vi "Main.vi"() -> ()   [LabVIEW 2016]
uses:
  Type Defs/Target.ctl
  Type Defs/Current Coords.ctl
  Type Defs/Host Data.ctl
panel:
  in  "kp":dbl=0.02
  in  "kd":dbl=0.001
  in  "ki":dbl=0.002
  in  "Disturbance":bool
  out "state":string
  out "Current Position":T1
  in  "Target":T2
  in  "stop":bool
  in  "Start":bool
  in  "Tab Control":enum32{"Arm Location", "Arm Coords"}(tab)
  out "Link Picture":picture
  out "Current arm location":cluster{"X":dbl, "Y":dbl}[](graph)=[{"X"=0.0, "Y"=0.0}, {"X"=4.2862637970157365e-15, "Y"=70.0}, {"X"=70.0, "Y"=70.0}]
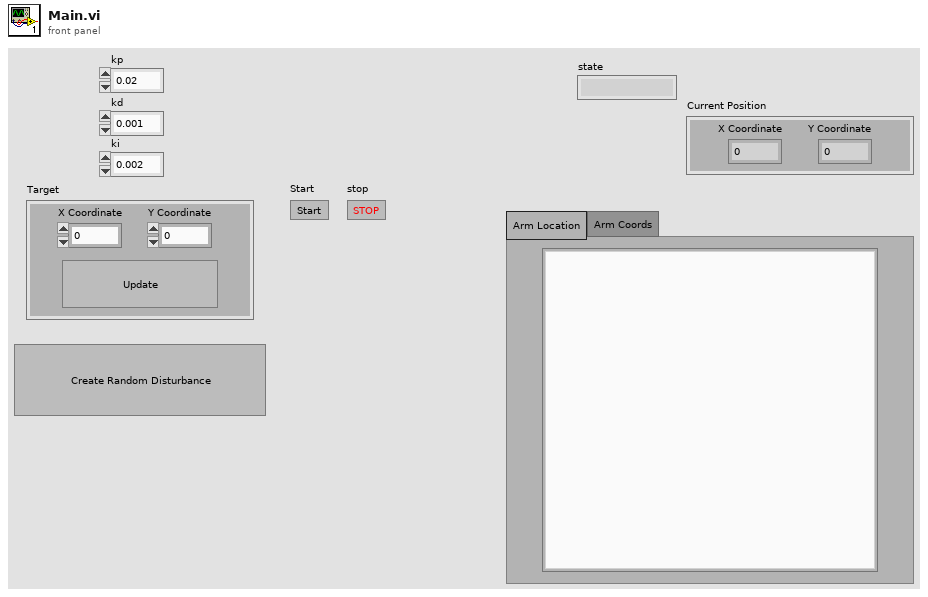
[diagram p1: front panel]
types:
  T1 = typedef "Current Coords.ctl" = cluster{"X Coordinate":dbl, "Y Coordinate":dbl}
  T2 = typedef "Target.ctl" = cluster{"X Coordinate":dbl, "Y Coordinate":dbl, "Update":bool}
  T3 = typedef "Host Data.ctl" = cluster{"link 1 angle":dbl, "link 2 angle":dbl, "link 1 length":dbl, "link 2 length":dbl, "Current arm location":cluster{"X":dbl, "Y":dbl}[], "Link Picture":picture, "Desired Location":cluster{"Desired X":dbl, "Desired Y":dbl}, "Next Location":cluster{"Next X":dbl, "Next Y":dbl}, "Error":cluster{"Joint1 error":dbl, "Joint2 error":dbl}, "tdms data":refnum<k34>, "de/dt":cluster{"joint1 de/dt":dbl, "joint2 de/dt":dbl}, "Voltages":cluster{"Joint1 voltage":dbl, "Joint2 voltage":dbl}, "Time":dbl, "dt":dbl, "counts/rev":dbl, "kp":dbl, "kd":dbl, "ki":dbl, "Int(error)":cluster{"joint1 int(e)":dbl, "joint2 int(e)":dbl}, "Desired angles":cluster{"theta 1":dbl, "theta 2":dbl}, "Current counts":cluster{"theta 1":dbl, "theta 2":dbl}, "Desired Counts":cluster{"theta 1":dbl, "theta 2":dbl}, "Preivous Error":cluster{"Joint1 Previous error":dbl, "Joint2 Previous error":dbl}, "Counts/s":dbl, "Correct counter":i32}
  T4 = enum8{"Enabled", "Disabled", "Disabled and Grayed Out"}
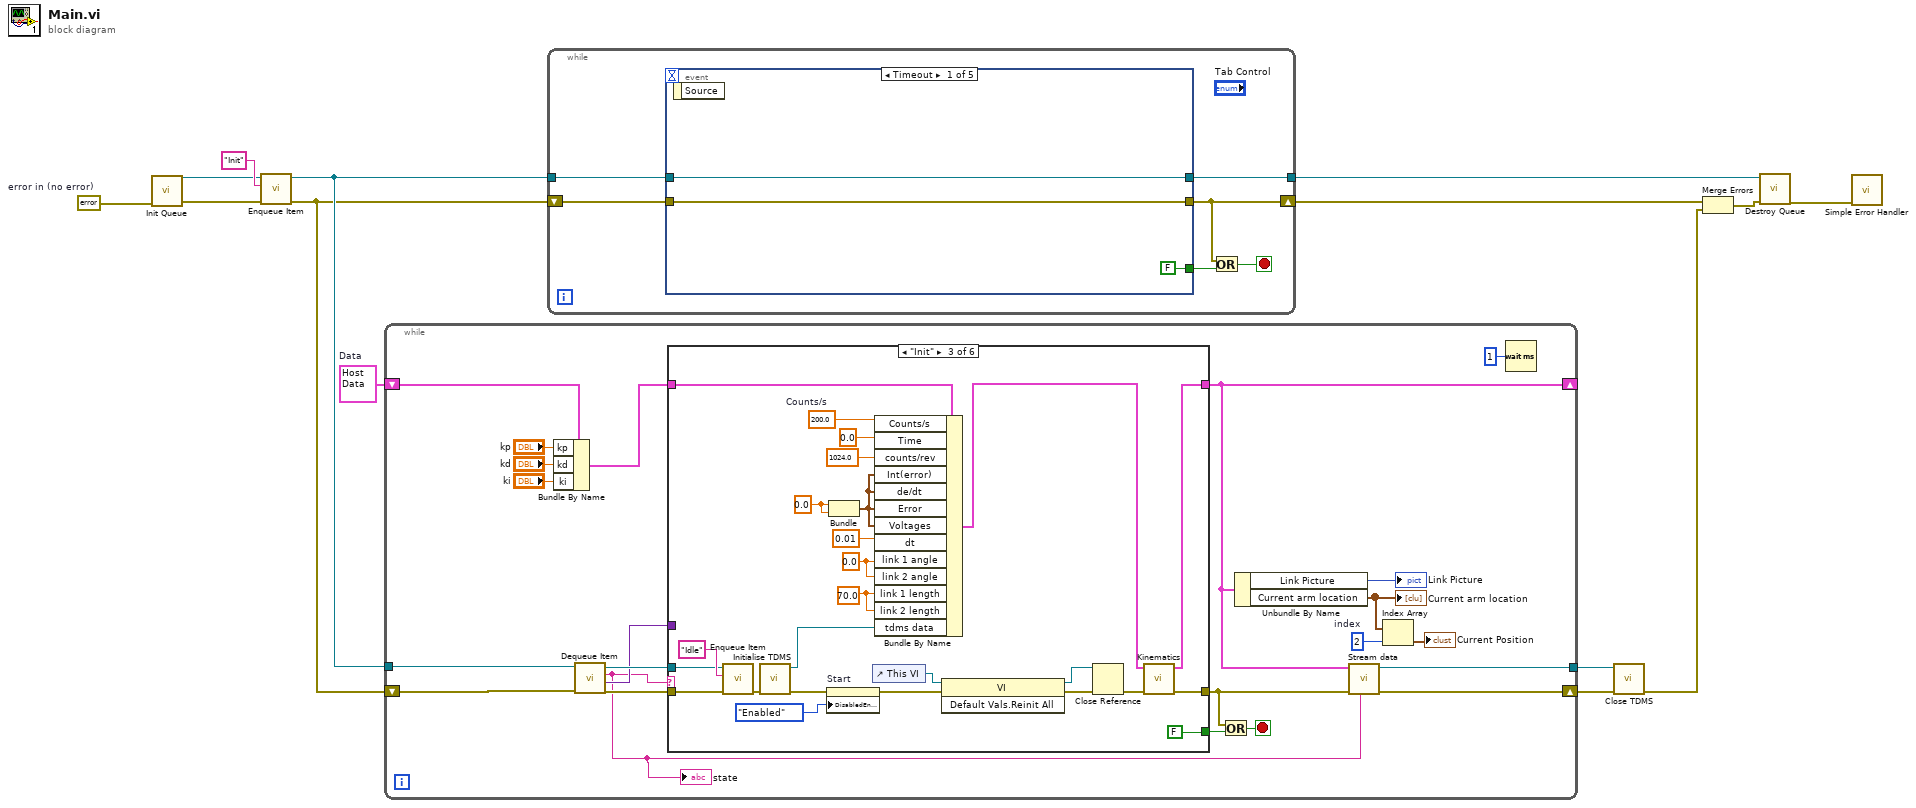
[diagram p0: block diagram]
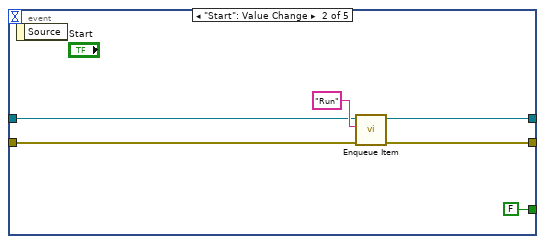
[diagram p2: hidden frame]
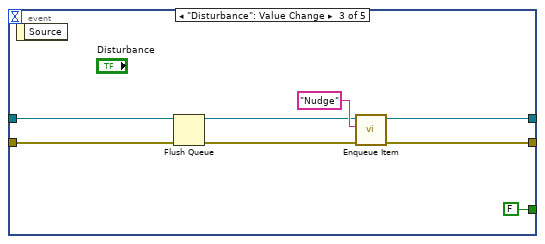
[diagram p3: hidden frame]
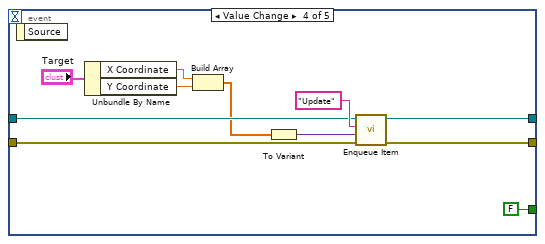
[diagram p4: hidden frame]
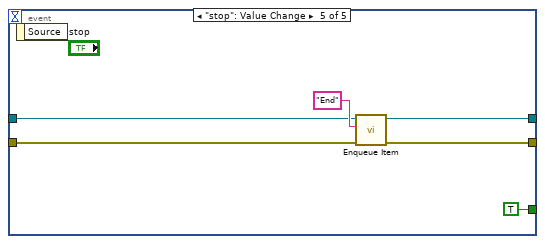
[diagram p5: hidden frame]
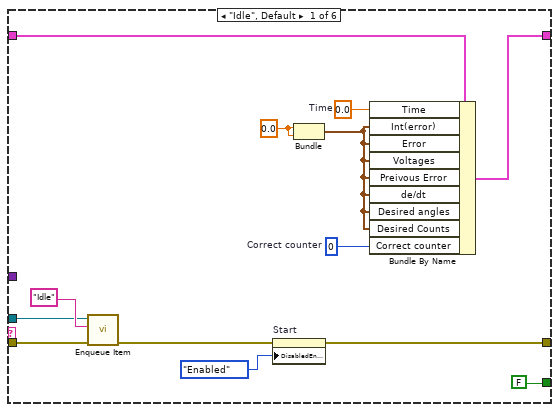
[diagram p6: hidden frame]
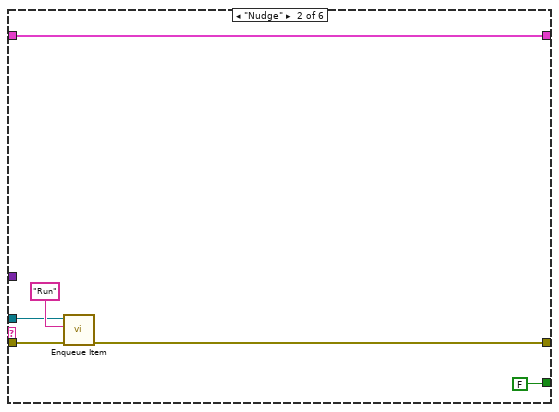
[diagram p7: hidden frame]
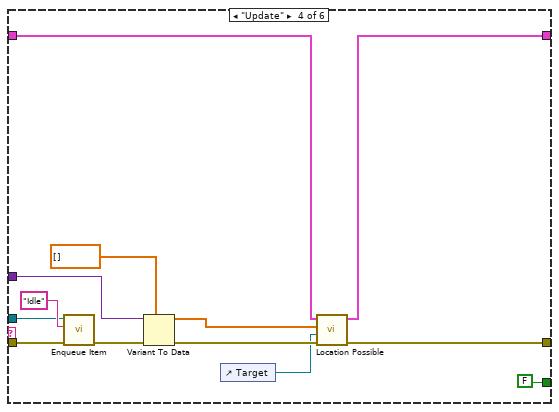
[diagram p8: hidden frame]
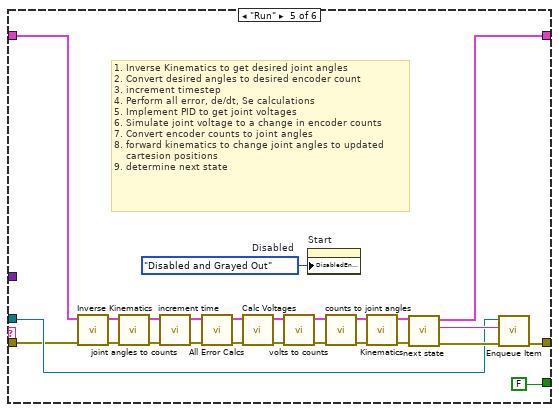
[diagram p9: hidden frame]
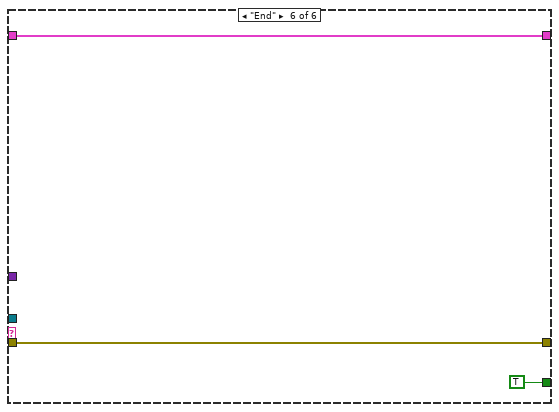
[diagram p10: hidden frame]
diagram:
  w10 = errorcluster {"status"=FALSE, "code"=0, "source"=""}  # error in (no error)
  w9 = T3 {"link 1 angle"=0.0, "link 2 angle"=0.0, "link 1 length"=0.0, "link 2 length"=0.0, "Current arm location"=[{"X"=0.0, "Y"=0.0}, {"X"=-37.249783598972314, "Y"=33.353464914904016}, {"X"=-74.49956719794463, "Y"=66.70692982980803}], "Link Picture"=bytes[1162], "Desired Location"={"Desired X"=0.0, "Desired Y"=0.0}, "Next Location"={"Next X"=0.0, "Next Y"=0.0}, "Error"={"Joint1 error"=0.0, "Joint2 error"=0.0}, "tdms data"=refnum, "de/dt"={"joint1 de/dt"=0.0, "joint2 de/dt"=0.0}, "Voltages"={"Joint1 voltage"=0.0, "Joint2 voltage"=0.0}, "Time"=0.0, "dt"=0.0, "counts/rev"=0.0, "kp"=0.0, "kd"=0.0, "ki"=0.0, "Int(error)"={"joint1 int(e)"=0.0, "joint2 int(e)"=0.0}, "Desired angles"={"theta 1"=0.0, "theta 2"=0.0}, "Current counts"={"theta 1"=0.0, "theta 2"=0.0}, "Desired Counts"={"theta 1"=0.0, "theta 2"=0.0}, "Preivous Error"={"Joint1 Previous error"=0.0, "Joint2 Previous error"=0.0}, "Counts/s"=0.0, "Correct counter"=0}  # Data
  n1 = call "Init Queue.vi"("error in (no error)"=w10) -> ("error out"=w11:errorcluster, "Queue out"=w12:refnum<queue>)  [unwired: 9 in]
  n2 = call "Enqueue Item.vi"("error in (no error)"=w11, "State"="Init", "Queue in"=w12) -> ("error out"=w4:errorcluster, "Queue out"=w13:refnum<queue>)  [unwired: 7 in]
  n3 = while {
    tunnel: w13 -> [w36]
    shift-right: [w23] -> w3
    shift-left: w4 -> [w35]
    shift-right: [w22] -> _
    shift-left: w9 -> [w19]
    tunnel: [w20] -> w1
    stop <- w31 stop-if-true
    w26 = 2  # index
    n4 = Bundle By Name(cluster=w19, "kp"="kp", "kd"="kd", "ki"="ki") -> (w18:T3)
    n5 = call "Dequeue Item.vi"("error in (no error)"=w35, "Queue in"=w36) -> ("error out"=w34:errorcluster, "Variant"=w32:variant, "String"=w21:string, "Queue out"=w33:refnum<queue>)  [unwired: 6 in]
    "state" <- w21
    n6 = case shown="\"Init\"" w21 {
      tunnel: w34 -> [w47 w53 w78 w88 w111 w121]
      tunnel: w33 -> [w46 w52 w77 w89 w113 _]
      tunnel: w32 -> [_ _ _ w93 _ _]
      tunnel: [w37 w50 w71 w81 w115 w121] -> w24
      tunnel: [FALSE FALSE FALSE FALSE FALSE TRUE] -> w30
      tunnel: w18 -> [w45 w51 w76 w85 w112 w119]
      tunnel: [w44 w51 w72 w82 w117 w119] -> w22
      frame "Idle", Default {
        w41 = 0.0 ("Time")
        w42 = 0  # Correct counter
        w43 = 0.0  # Time
        n7 = call "Enqueue Item.vi"("error in (no error)"=w47, "State"="Idle", "Queue in"=w46) -> ("error out"=w38:errorcluster)  [unwired: 7 in, 1 out]
        n8 = property on="Start" class="Bool"(error in=w38, "DisabledEnum"=T4."Enabled" ("Disabled")) -> (error out=w37:errorcluster)  [unwired: 1 in, 1 out]
        n9 = Bundle("Time"=w41, "Time"=w41) -> (w40:cluster{"Time":dbl, "Time":dbl})  [unwired: 1 in]
        n10 = Bundle By Name(cluster=w45, "Time"=w43, "Int(error)"=w40, "Error"=w40, "Voltages"=w40, "Preivous Error"=w40, "de/dt"=w40, "Desired angles"=w40, "Desired Counts"=w40, "Correct counter"=w42) -> (w44:T3)
      }
      frame "Nudge" {
        n11 = call "Enqueue Item.vi"("error in (no error)"=w53, "State"="Run", "Queue in"=w52) -> ("error out"=w50:errorcluster)  [unwired: 7 in, 1 out]
      }
      frame "Init" {
        w59 = 200.0  # Counts/s
        w64 = 0.0
        w74 = 70.0
        w75 = 0.0
        n12 = call "Enqueue Item.vi"("error in (no error)"=w78, "State"="Idle", "Queue in"=w77) -> ("error out"=w66:errorcluster)  [unwired: 7 in, 1 out]
        n13 = call "Initialise TDMS.vi"("error in (no error)"=w66) -> ("error out"=w57:errorcluster, "tdms file out"=w65:refnum<k34>)  [unwired: 9 in]
        n14 = property on="Start" class="Bool"(error in=w57, "DisabledEnum"=T4."Enabled" ("Disabled")) -> (error out=w56:errorcluster)  [unwired: 1 in, 1 out]
        n15 = Bundle(w64, w64) -> (w62:cluster{dbl, dbl})  [unwired: 1 in]
        n16 = control-ref of="This VI"() -> (w70:refnum<vi>)
        n17 = Bundle By Name(cluster=w76, "Counts/s"=w59, "Time"=0.0, "counts/rev"=1024.0, "Int(error)"=w62, "de/dt"=w62, "Error"=w62, "Voltages"=w62, "dt"=0.01, "link 1 angle"=w75, "link 2 angle"=w75, "link 1 length"=w74, "link 2 length"=w74, "tdms data"=w65) -> (w73:T3)
        n18 = invoke class="VI" method="Default Vals.Reinit All"(reference=w70, error in=w56) -> (reference out=w67:refnum<vi>, error out=w69:errorcluster)  [unwired: 1 in, 1 out]
        n19 = Close Reference(reference=w67, error in (no error)=w69) -> (error out=w68:errorcluster)
        n20 = call "Kinematics.vi"("error in (no error)"=w68, "Data In"=w73) -> ("error out"=w71:errorcluster, "Data Out"=w72:T3)  [unwired: 8 in]
      }
      frame "Update" {
        n21 = call "Enqueue Item.vi"("error in (no error)"=w88, "State"="Idle", "Queue in"=w89) -> ("error out"=w87:errorcluster)  [unwired: 7 in, 1 out]
        n22 = Variant To Data(error in=w87, type=dbl[] [], Variant=w93) -> (data=w84:dbl[], error out=w86:errorcluster)
        n23 = control-ref of="Target"() -> (w83:refnum<vi>)
        n24 = call "Location Possible.vi"("error in (no error)"=w86, "Target"=w83, "Desired Location"=w84, "Data In"=w85) -> ("error out"=w81:errorcluster, "Data Out"=w82:T3)  [unwired: 6 in]
      }
      frame "Run" {
        w94 = T4."Disabled and Grayed Out"  # Disabled
        # "1. Inverse Kinematics to get desired joint angles\n2. Convert desired angles to desired encoder count\n3. increment timestep\n4. Perform all error, de/dt, Se calculations\n5. Implement PID to get joint voltages\n6. Simulate joint voltage to a change in encoder counts\n7. Convert encoder counts to joint angles\n8. forward kinematics to change joint angles to updated\n    cartesion positions\n9. determine next state"
        n25 = call "Inverse Kinematics.vi"("error in (no error)"=w111, "Data in"=w112) -> ("error out"=w109:errorcluster, "Data Out"=w110:T3)  [unwired: 8 in]
        n26 = call "joint angles to counts.vi"("error in (no error)"=w109, "Data in"=w110) -> ("error out"=w107:errorcluster, "Data out"=w108:T3)  [unwired: 8 in]
        n27 = call "increment time.vi"("error in (no error)"=w107, "Data in"=w108) -> ("error out"=w105:errorcluster, "Data Out"=w106:T3)  [unwired: 8 in]
        n28 = call "All Error Calcs.vi"("error in (no error)"=w105, "Data in"=w106) -> ("error out"=w103:errorcluster, "Data Out"=w104:T3)  [unwired: 8 in]
        n29 = call "Calc Voltages.vi"("error in (no error)"=w103, "Data In"=w104) -> ("error out"=w101:errorcluster, "Data Out"=w102:T3)  [unwired: 8 in]
        n30 = call "volts to counts.vi"("error in (no error)"=w101, "Data In"=w102) -> ("error out"=w99:errorcluster, "Data Out"=w100:T3)  [unwired: 8 in]
        n31 = property on="Start" class="Bool"("DisabledEnum"=w94) -> ()  [unwired: 2 in, 2 out]
        n32 = call "counts to joint angles.vi"("error in (no error)"=w99, "Data in"=w100) -> ("error out"=w97:errorcluster, "Data out"=w98:T3)  [unwired: 8 in]
        n33 = call "Kinematics.vi"("error in (no error)"=w97, "Data In"=w98) -> ("error out"=w95:errorcluster, "Data Out"=w96:T3)  [unwired: 8 in]
        n34 = call "next state.vi"("error in (no error)"=w95, "Data in"=w96) -> ("error out"=w116:errorcluster, "Next State"=w114:string, "Data out"=w117:T3)  [unwired: 7 in]
        n35 = call "Enqueue Item.vi"("error in (no error)"=w116, "State"=w114, "Queue in"=w113) -> ("error out"=w115:errorcluster)  [unwired: 7 in, 1 out]
      }
      frame "End" {
      }
    }
    n36 = Or(x=w24, y=w30) -> (x .or. y?=w31:bool)
    n37 = Unbundle By Name(w22) -> ("Link Picture"=→"Link Picture":picture, "Current arm location"=w27:cluster{"X":dbl, "Y":dbl}[])
    "Current arm location" <- w27
    n38 = call "Stream data.vi"("state"=w21, "error in (no error)"=w24, "Data"=w22) -> ("error out"=w23:errorcluster, "tdms file out"=w20:refnum<k34>)  [unwired: 7 in]
    n39 = Index Array(array=w27, index=w26) -> (element=→"Current Position":cluster{"X":dbl, "Y":dbl})
    n40 = Wait (ms)(milliseconds to wait=u32 1) -> ()  [unwired: 1 out]
  }
  n41 = while {
    shift-right: [w125] -> w6
    shift-left: w4 -> [w127]
    tunnel: w13 -> [w123]
    tunnel: [w122] -> w8
    stop <- w126 stop-if-true
    n42 = event shown="[0] Timeout" {
      selector: _ -> [_ _ _ _ _]
      dyn-events: _ -> [_ _ _ _ _]
      timeout: _ -> [_ _ _ _ _]
      tunnel: w127 -> [w130 w135 w138 w154 w161]
      tunnel: [w130 w136 w144 w155 w160] -> w125
      tunnel: [FALSE FALSE FALSE FALSE TRUE] -> w124
      tunnel: w123 -> [w128 w132 w140 w151 w157]
      tunnel: [w128 w131 w141 w145 w156] -> w122
      event Timeout {
        n43 = event-data() -> ()  [unwired: 1 in, 1 out]
      }
      event "Start": Value Change {
        n44 = event-data() -> ()  [unwired: 1 in, 1 out]
        n45 = call "Enqueue Item.vi"("error in (no error)"=w135, "State"="Run", "Queue in"=w132) -> ("error out"=w136:errorcluster, "Queue out"=w131:refnum<queue>)  [unwired: 7 in]
      }
      event "Disturbance": Value Change {
        n46 = event-data() -> ()  [unwired: 1 in, 1 out]
        n47 = Flush Queue(queue=w140, error in (no error)=w138) -> (queue out=w139:refnum<queue>, error out=w137:errorcluster)  [unwired: 1 out]
        n48 = call "Enqueue Item.vi"("error in (no error)"=w137, "State"="Nudge", "Queue in"=w139) -> ("error out"=w144:errorcluster, "Queue out"=w141:refnum<queue>)  [unwired: 7 in]
      }
      event Value Change {
        n49 = event-data() -> ()  [unwired: 1 in, 1 out]
        n50 = Unbundle By Name("Target") -> ("X Coordinate"=w148:dbl, "Y Coordinate"=w149:dbl)
        n51 = Build Array(w148, w149) -> (w147:dbl[])
        n52 = To Variant(anything=w147) -> (Variant=w146:variant)
        n53 = call "Enqueue Item.vi"("error in (no error)"=w154, "Message"=w146, "State"="Update", "Queue in"=w151) -> ("error out"=w155:errorcluster, "Queue out"=w145:refnum<queue>)  [unwired: 6 in]
      }
      event "stop": Value Change {
        n54 = event-data() -> ()  [unwired: 1 in, 1 out]
        n55 = call "Enqueue Item.vi"("error in (no error)"=w161, "State"="End", "Queue in"=w157) -> ("error out"=w160:errorcluster, "Queue out"=w156:refnum<queue>)  [unwired: 7 in]
      }
    }
    n56 = Or(x=w125, y=w124) -> (x .or. y?=w126:bool)
  }
  n57 = call "Close TDMS.vi"("error in (no error)"=w3, "tdms file"=w1) -> ("error out"=w2:errorcluster)  [unwired: 9 in]
  n58 = Merge Errors(w6, w2) -> (w5:errorcluster)
  n59 = call "Destroy Queue.vi"("error in (no error)"=w5, "Queue in"=w8) -> ("error out"=w7:errorcluster)  [unwired: 9 in]
  n60 = call <vilib>:"Simple Error Handler.vi"("error in (no error)"=w7) -> ()  [unwired: 4 in, 5 out]
